vi "LookForParentPhaseCalc.vi"(6 "calc cache in":variant, 7 "feature name":string, 9 "channel name":string, 10 "pulse positions":dbl[](array[numeric]), 11 "waveform to use in phase band calculation":waveform(sgl)) -> (1 "parent channel phase value":dbl, 2 "found cached parent phase":bool, 3 "Cross phase [degrees]":cluster{"f0":dbl, "df":dbl, "phase":sgl[]}, 4 "calc cache out":variant)   [LabVIEW 2017, in "AnalysisHelper.lvlib"]
uses:
  <vilib>/addons/InsightCM/Utilities/Analysis/Shared/AnalysisHelper.lvlib
  <vilib>/addons/InsightCM/Utilities/Analysis/Vibration/VibrationAnalysisFunctions.lvlib
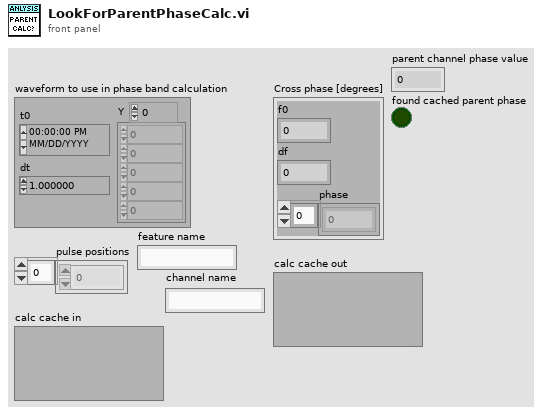
[diagram p1: front panel]
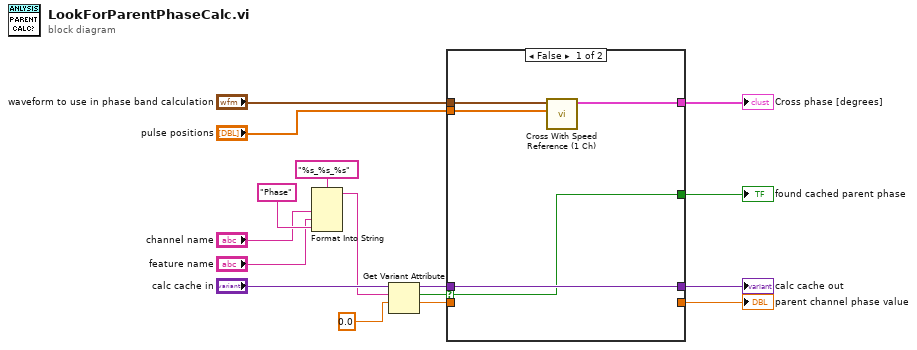
[diagram p0: block diagram]
diagram:
  n1 = Format Into String(format string="%s_%s_%s", "channel name", "feature name", "Phase" ("name")) -> (resulting string=w8:string)  [unwired: 2 in, 1 out]
  n2 = Get Variant Attribute(Variant="calc cache in", name=w8, default value (empty Variant)=0.0 ("phase")) -> (duplicate Variant=w2:variant, found=w6:bool, value=w5:dbl)  [unwired: 1 in, 1 out]
  n3 = case shown="False" w6 {
    selector: w6 -> [w17 w22]
    tunnel: [w21 _] -> w16
    tunnel: "pulse positions" -> [w20 _]
    tunnel: "waveform to use in phase band calculation" -> [w19 _]
    tunnel: w5 -> [_ w24]
    tunnel: [_ w24] -> w4
    tunnel: [w18 w23] -> w3
    tunnel: w2 -> [w18 w23]
    tunnel: [w17 w22] -> w1
    frame False {
      n4 = call <vilib>:"Cross With Speed Reference (1 Ch).vi"("Speed Profile (Positions [s])"=w20, "Waveform"=w19) -> ("Cross phase [degrees]"=w21:cluster{"f0":dbl, "df":dbl, "phase":sgl[]})  [unwired: 8 in, 1 out]
    }
    frame True {
    }
  }
  "calc cache out" <- w3
  "Cross phase [degrees]" <- w16
  "parent channel phase value" <- w4
  "found cached parent phase" <- w1
